vi "align selection.vi"(7 "main-national data":T1={"board vision"=[["green", "", "", ""], ["black", "", "", ""], ["", "", "", "yellow"], ["blue", "", "", ""], ["red", "", "", ""]], "recycle room"=[], "box array"=[], "catch array"=[], "put room"="", "catch count"=0.0, "position set"={"vision board"=0.0, "catch box"=0.0, "R1 position"=0.0, "R5 position"=0.0}, "reg data"=[], "S gyro"=0.0}, 8 "error in (no error)":errorcluster, 11 "align type":T4) -> (0 "error out":errorcluster, 1 "Position":T3, 3 "main-national data out":T1={"board vision"=[["green", "", "", ""], ["black", "", "", ""], ["", "", "", "yellow"], ["blue", "", "", ""], ["red", "", "", ""]], "recycle room"=[], "box array"=[], "catch array"=[], "put room"="", "catch count"=0.0, "position set"={"vision board"=0.0, "catch box"=0.0, "R1 position"=0.0, "R5 position"=0.0}, "reg data"=[], "S gyro"=0.0})   [LabVIEW 2019]
uses:
  ctl/align type.ctl
  subVI/move/position cluster.ctl
  ctl/main data-national.ctl
  ctl/position set.ctl
  ctl/height.ctl
  ctl/servo act.ctl
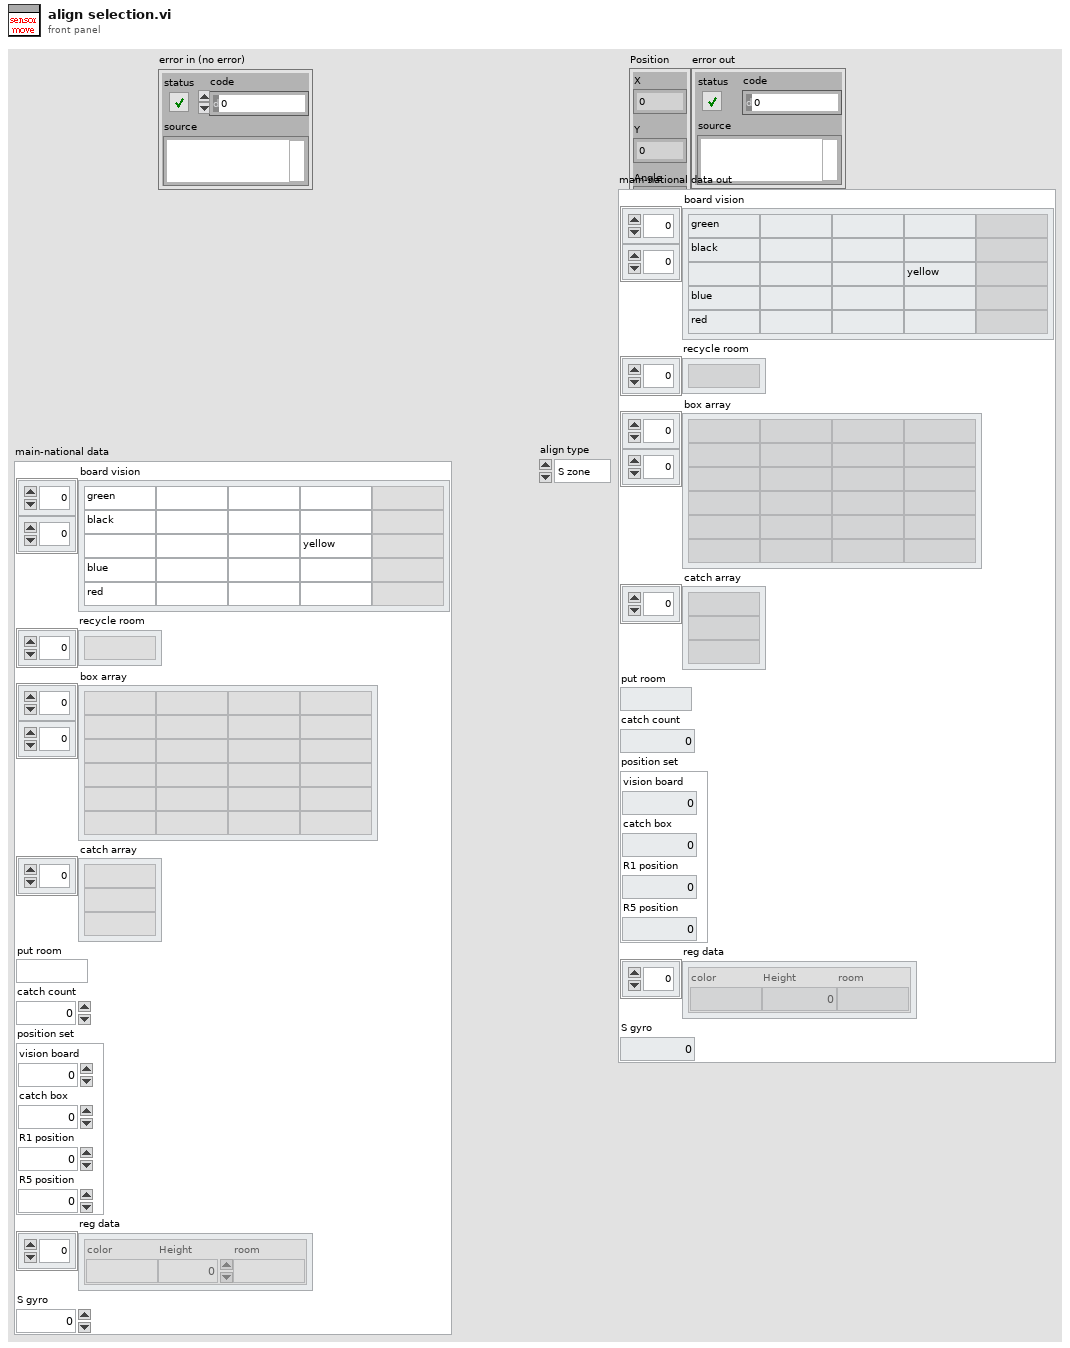
[diagram p1: front panel]
types:
  T1 = typedef "main data-national.ctl" = cluster{"board vision":string[][], "recycle room":string[], "box array":string[][], "catch array":string[], "put room":string, "catch count":dbl, "position set":T2, "reg data":cluster{"color":string, "Height":i32, "room":string}[], "S gyro":dbl}
  T2 = typedef "position set.ctl" = cluster{"vision board":dbl, "catch box":dbl, "R1 position":dbl, "R5 position":dbl}
  T3 = typedef "position cluster.ctl" = cluster{"X":dbl, "Y":dbl, "Angle":dbl}
  T4 = typedef "align type.ctl" = enum16{"S zone", "box align", "box align contrast", "R1 align", "R5 align", "-> R5 center align", "-> R1 center align"}
  T5 = typedef "servo act.ctl" = enum16{"catch", "relax", "left idle", "center", "red relax", "left reg", "right reg"}
  T6 = typedef "height.ctl" = enum16{"IDLE", "recycle pre-catch", "recycle catch", "recycle zone", "vision height", "box 1", "box 2", "box 3", "box 1 pre", "box 2 pre", "box 3 pre", "reg 1", "reg 2", "reg 1 pre", "reg 2 pre", "put 1", "put 2", "put 3"}
  T7 = typedef "BNO055 gyro 3axis.ctl" = cluster{"yaw":dbl, "pitch":dbl, "roll":dbl}
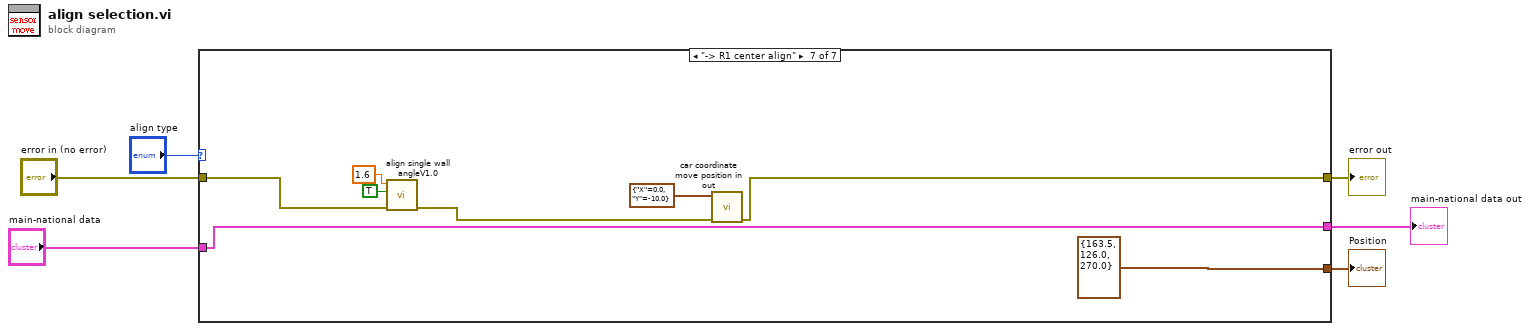
[diagram p0: block diagram]
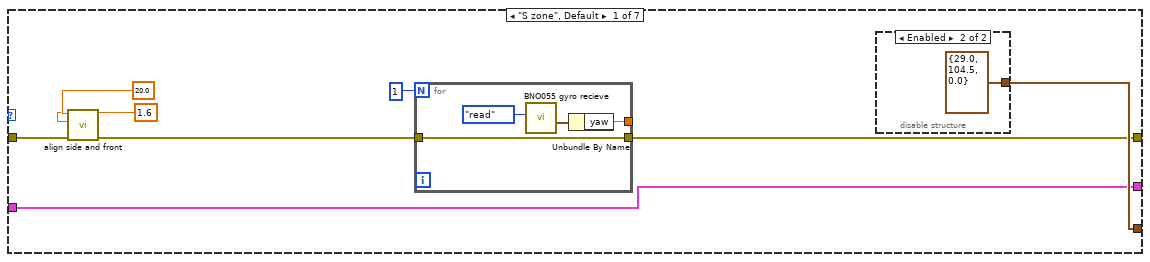
[diagram p2: hidden frame]
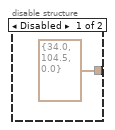
[diagram p3: hidden frame]
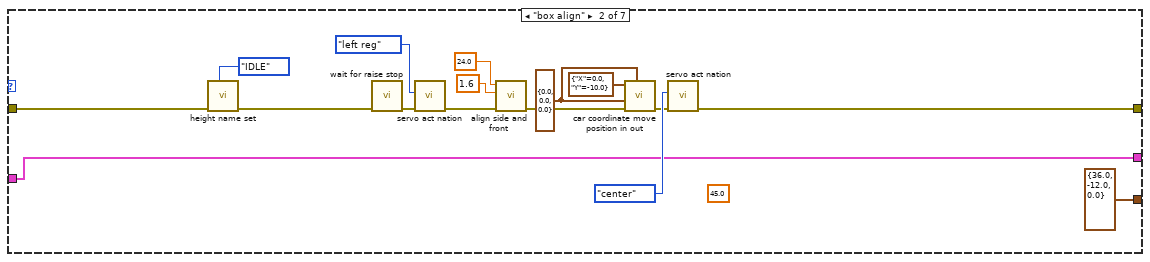
[diagram p4: hidden frame]
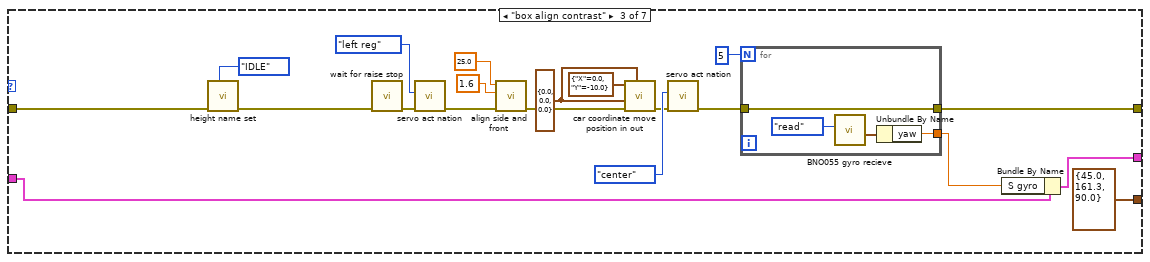
[diagram p5: hidden frame]
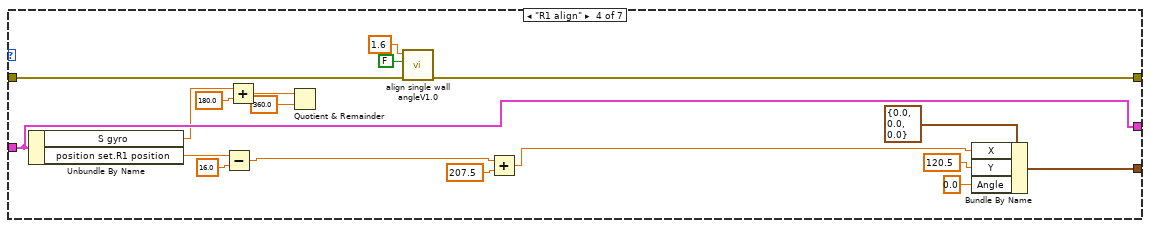
[diagram p6: hidden frame]
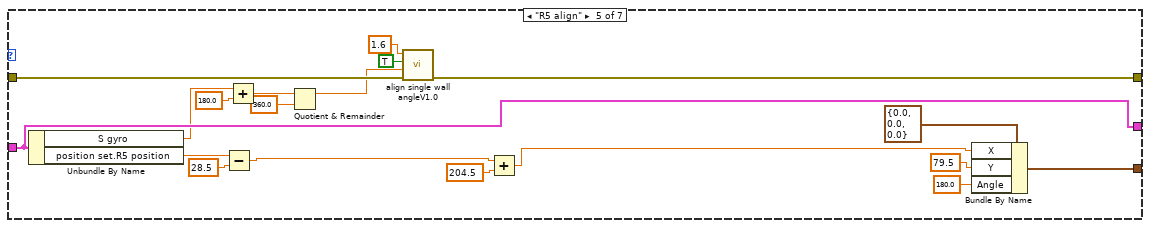
[diagram p7: hidden frame]
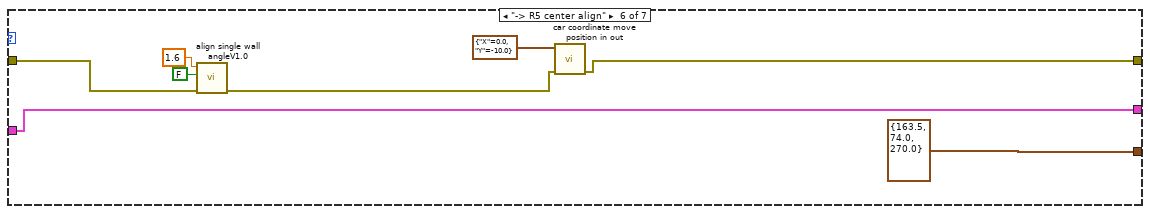
[diagram p8: hidden frame]
diagram:
  n1 = case shown="\"-> R1 center align\"" "align type" {
    tunnel: [w14 T3 {"X"=36.0, "Y"=-12.0, "Angle"=0.0} ("Position") T3 {"X"=45.0, "Y"=161.3, "Angle"=90.0} ("Position") w75 w94 T3 {"X"=163.5, "Y"=74.0, "Angle"=270.0} ("Position") T3 {"X"=163.5, "Y"=126.0, "Angle"=270.0} ("Position")] -> w5
    tunnel: [w9 w23 w40 w76 w95 w99 w106] -> w4
    tunnel: "error in (no error)" -> [w13 w24 w53 w77 w96 w103 w111]
    tunnel: "main-national data" -> [w8 w22 w39 w72 w91 w102 w110]
    tunnel: [w8 w22 w38 w72 w91 w102 w110] -> w1
    frame "S zone", Default {
      n2 = call "align side and front.vi"("error in (no error)"=w13, "Target (Volt)"=1.6, "Setpoint"=20.0) -> ("error out"=w10:errorcluster)  [unwired: 8 in]
      n3 = for {
        N: 1 -> [_]
        tunnel: w10 -> [w18]
        tunnel: [w18] -> w9
        tunnel: [w15] -> _
        n4 = call "BNO055 gyro recieve.vi"("Enum"=enum16{"read", "write"}."read") -> ("read"=w16:T7)  [unwired: 10 in]
        n5 = Unbundle By Name(w16) -> ("yaw"=w15:dbl)
      }
      n6 = disable-structure shown="Enabled" {
        disable-tunnel: [T3 {"X"=34.0, "Y"=104.5, "Angle"=0.0} ("Position") T3 {"X"=29.0, "Y"=104.5, "Angle"=0.0} ("Position")] -> w14
        frame Disabled {
        }
        frame Enabled {
        }
      }
    }
    frame "box align" {
      w21 = T3 {"X"=0.0, "Y"=0.0, "Angle"=0.0} ("Position in")
      (unwired) 45.0 ("speed")
      n7 = call "height name set.vi"("height name"=height."IDLE", "error in (no error)"=w24) -> ("error out"=w32:errorcluster)  [unwired: 9 in]
      n8 = call "wait for raise stop.vi"("Error In"=w32) -> ("Error Out"=w31:errorcluster)  [unwired: 10 in]
      n9 = call "servo act nation.vi"("error in"=w31, "servo act"=servo_act."left reg") -> ("error out"=w29:errorcluster)  [unwired: 9 in]
      n10 = call "align side and front.vi"("error in (no error)"=w29, "Target (Volt)"=1.6, "Setpoint"=24.0) -> ("error out"=w27:errorcluster)  [unwired: 8 in]
      n11 = call "car coordinate move position in out.vi"("Position in 2"=w21, "error in (no error)"=w27, "Position in"=w21, "move"=cluster{"X":dbl, "Y":dbl} {"X"=0.0, "Y"=-10.0}) -> ("error out"=w25:errorcluster)  [unwired: 6 in, 1 out]
      n12 = call "servo act nation.vi"("error in"=w25, "servo act"=servo_act."center") -> ("error out"=w23:errorcluster)  [unwired: 9 in]
    }
    frame "box align contrast" {
      w37 = T3 {"X"=0.0, "Y"=0.0, "Angle"=0.0} ("Position in")
      n13 = call "height name set.vi"("height name"=height."IDLE", "error in (no error)"=w53) -> ("error out"=w51:errorcluster)  [unwired: 9 in]
      n14 = call "wait for raise stop.vi"("Error In"=w51) -> ("Error Out"=w50:errorcluster)  [unwired: 10 in]
      n15 = call "servo act nation.vi"("error in"=w50, "servo act"=servo_act."left reg") -> ("error out"=w48:errorcluster)  [unwired: 9 in]
      n16 = call "align side and front.vi"("error in (no error)"=w48, "Target (Volt)"=1.6, "Setpoint"=25.0) -> ("error out"=w46:errorcluster)  [unwired: 8 in]
      n17 = call "car coordinate move position in out.vi"("Position in 2"=w37, "error in (no error)"=w46, "Position in"=w37, "move"=cluster{"X":dbl, "Y":dbl} {"X"=0.0, "Y"=-10.0}) -> ("error out"=w44:errorcluster)  [unwired: 6 in, 1 out]
      n18 = call "servo act nation.vi"("error in"=w44, "servo act"=servo_act."center") -> ("error out"=w41:errorcluster)  [unwired: 9 in]
      n19 = for {
        N: 5 -> [_]
        tunnel: w41 -> [w60]
        tunnel: [w60] -> w40
        tunnel: [w57] -> w42
        n20 = call "BNO055 gyro recieve.vi"("Enum"=enum16{"read", "write"}."read") -> ("read"=w58:T7)  [unwired: 10 in]
        n21 = Unbundle By Name(w58) -> ("yaw"=w57:dbl)
      }
      n22 = Bundle By Name(cluster=w39, "S gyro"=w42) -> (w38:T1)
    }
    frame "R1 align" {
      n23 = Unbundle By Name(w72) -> ("S gyro"=w71:dbl, "position set.R1 position"=w70:dbl)
      n24 = Subtract(x=w70, y=16.0) -> (x-y=w68:dbl)
      n25 = Add(x=w71, y=180.0) -> (x+y=w64:dbl)
      n26 = Quotient & Remainder(x=w64, y=360.0) -> ()  [unwired: 2 out]
      n27 = call "align single wall angleV1.0.vi"("error in (no error)"=w77, "dir"=FALSE, "Target Voltage"=1.6) -> ("Error Out"=w76:errorcluster)  [unwired: 8 in]
      n28 = Add(x=w68, y=207.5) -> (x+y=w66:dbl)
      n29 = Bundle By Name(cluster=T3 {"X"=0.0, "Y"=0.0, "Angle"=0.0} ("Position"), "X"=w66, "Y"=120.5, "Angle"=0.0) -> (w75:T3)
    }
    frame "R5 align" {
      n30 = Unbundle By Name(w91) -> ("S gyro"=w90:dbl, "position set.R5 position"=w89:dbl)
      n31 = Subtract(x=w89, y=28.5) -> (x-y=w87:dbl)
      n32 = Add(x=w90, y=180.0) -> (x+y=w83:dbl)
      n33 = Quotient & Remainder(x=w83, y=360.0) -> (x-y*floor(x/y)=w81:dbl)  [unwired: 1 out]
      n34 = call "align single wall angleV1.0.vi"("error in (no error)"=w96, "gyro degree"=w81, "dir"=TRUE, "Target Voltage"=1.6) -> ("Error Out"=w95:errorcluster)  [unwired: 7 in]
      n35 = Add(x=w87, y=204.5) -> (x+y=w85:dbl)
      n36 = Bundle By Name(cluster=T3 {"X"=0.0, "Y"=0.0, "Angle"=0.0} ("Position"), "X"=w85, "Y"=79.5, "Angle"=180.0) -> (w94:T3)
    }
    frame "-> R5 center align" {
      n37 = call "align single wall angleV1.0.vi"("error in (no error)"=w103, "dir"=FALSE, "Target Voltage"=1.6) -> ("Error Out"=w100:errorcluster)  [unwired: 8 in]
      n38 = call "car coordinate move position in out.vi"("error in (no error)"=w100, "move"=cluster{"X":dbl, "Y":dbl} {"X"=0.0, "Y"=-10.0}) -> ("error out"=w99:errorcluster)  [unwired: 8 in, 1 out]
    }
    frame "-> R1 center align" {
      n39 = call "align single wall angleV1.0.vi"("error in (no error)"=w111, "dir"=TRUE, "Target Voltage"=1.6) -> ("Error Out"=w107:errorcluster)  [unwired: 8 in]
      n40 = call "car coordinate move position in out.vi"("error in (no error)"=w107, "move"=cluster{"X":dbl, "Y":dbl} {"X"=0.0, "Y"=-10.0}) -> ("error out"=w106:errorcluster)  [unwired: 8 in, 1 out]
    }
  }
  "Position" <- w5
  "error out" <- w4
  "main-national data out" <- w1
